vi "Painting_Trajactory_Defalut.vi"(8 "Max-Min Voltage":cluster{"max":dbl, "min":dbl}, 10 "dt":dbl) -> (2 "Waveforms":waveform(dbl)[](graph))   [LabVIEW 2013]
doc: "图片控件可作为用户的绘图界面。本范例主要使用了画笔宽度和样式属性以及子集获取功能。子集获取是指从任意图像中截取一个矩形区域并绘制新图像的功能。"
uses:
  <vilib>/Utility/cursorutil.llb/Set Cursor (Icon Pict).vi
panel:
  in  "清除":bool
  in  "画笔颜色":u32(colorbox)
  in  "停止":bool
  in  "操作":u16(ring)=1 items=["绘制散点", "绘制自由格式线", "绘制直线", "绘制矩形", "选择子集"]
  out "子集":picture
  in  "选择画笔属性":T1={"宽度"=2, "样式"=enum."Solid"}
  out "图片":picture
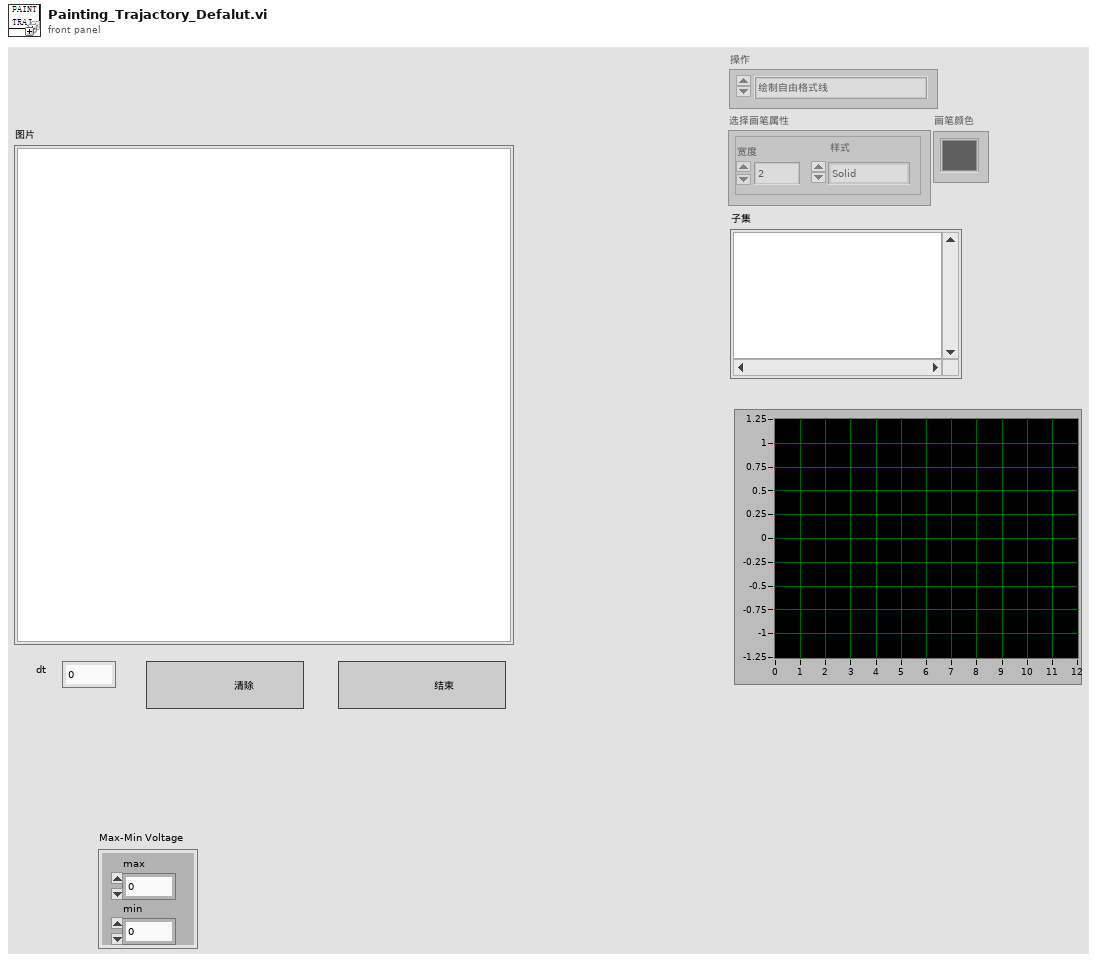
[diagram p1: front panel]
types:
  T1 = cluster{"宽度":u16, "样式":enum32{"Solid", "Dash", "Dot", "DashDot", "DashDotDot"}}
  T2 = enum32{"Solid", "Dash", "Dot", "DashDot", "DashDotDot"}
  T3 = cluster{"Width":u16, "Style":enum32{"Solid", "Dash", "Dot", "DashDot", "DashDotDot"}}
  T4 = enum8{"Enabled", "Disabled", "Disabled and Grayed Out"}
  T5 = typedef "LVMouseTypeDef.ctl" = cluster{"Mouse Position":cluster{"X":i32, "Y":i32}, "Mouse Modifiers":cluster{"Button Down":bool, "Shift Mod":bool, "Menu Mod":bool, "Option Mod":bool}}
  T6 = typedef "imagedata.ctl" = cluster{"image type":i32, "image depth":i32, "image":u8[], "mask":u8[], "colors":u32[], "Rectangle":cluster{"left":i16, "top":i16, "right":i16, "bottom":i16}}
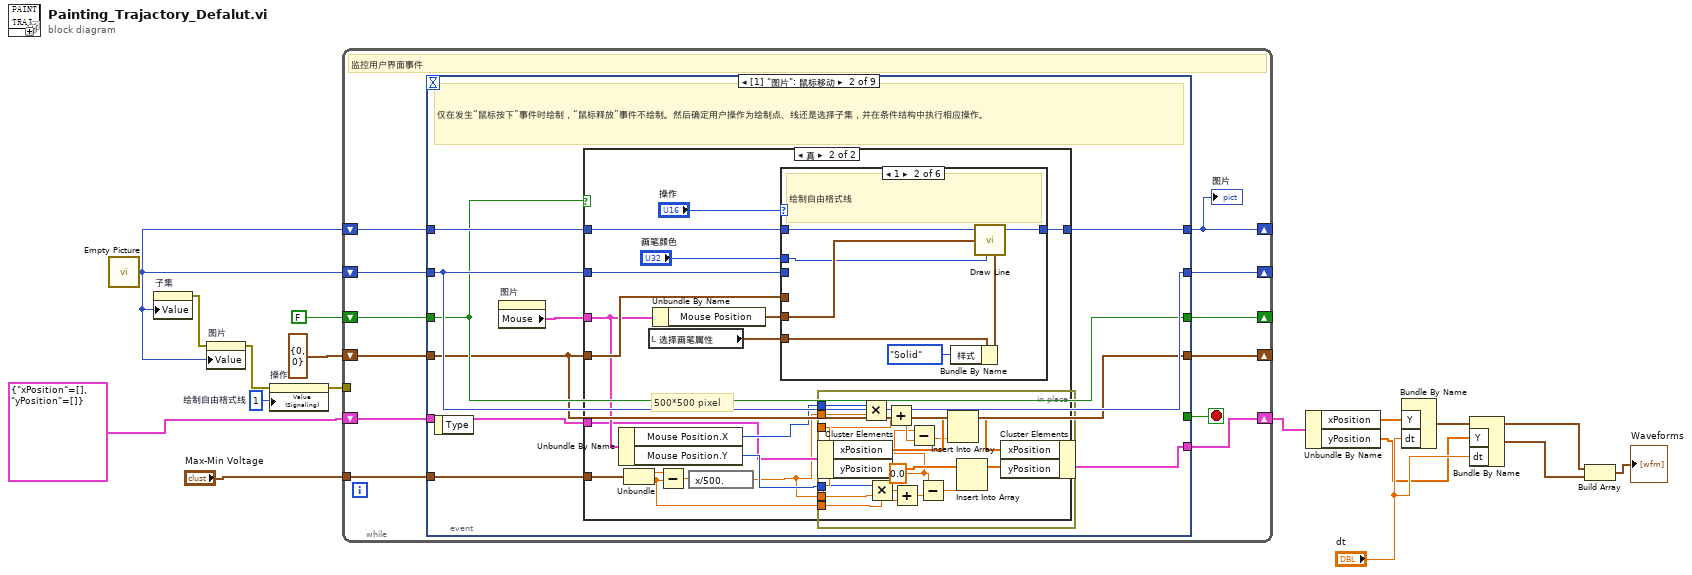
[diagram p0: block diagram]
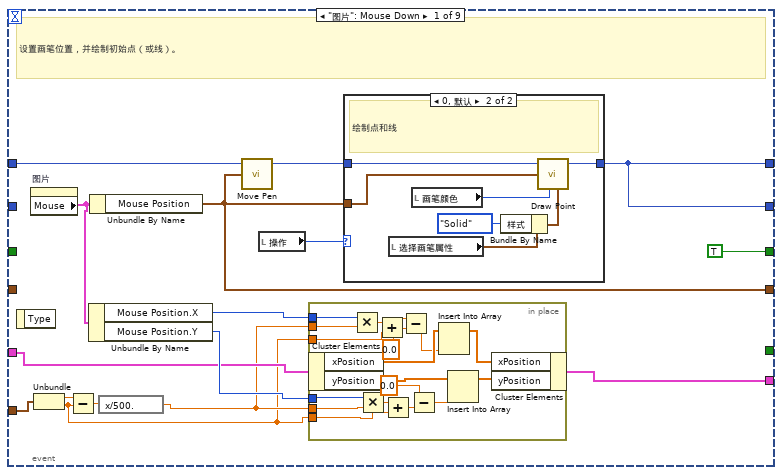
[diagram p2: hidden frame]
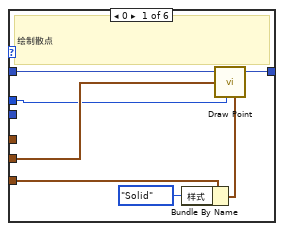
[diagram p5: hidden frame]
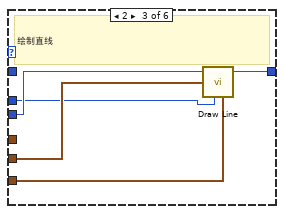
[diagram p6: hidden frame]
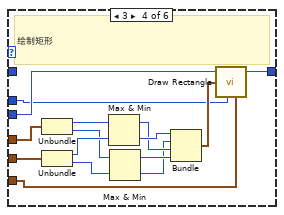
[diagram p7: hidden frame]
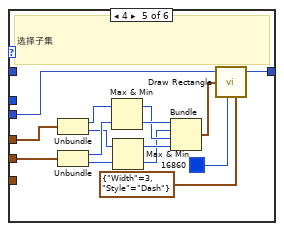
[diagram p8: hidden frame]
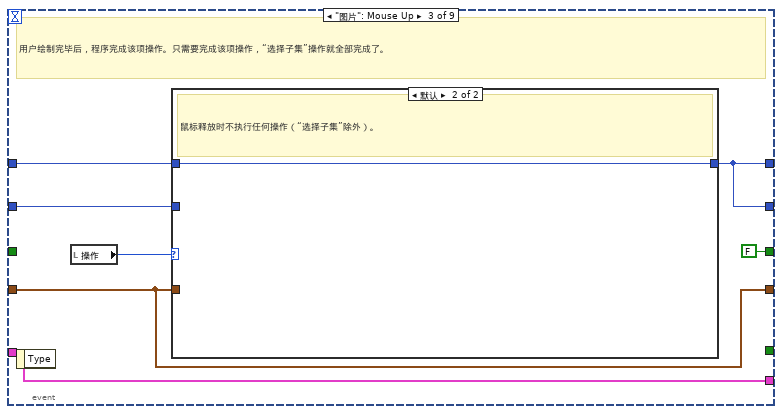
[diagram p10: hidden frame]
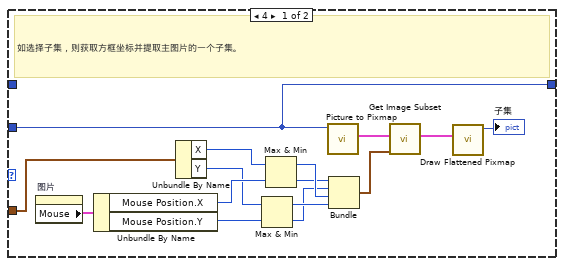
[diagram p11: hidden frame]
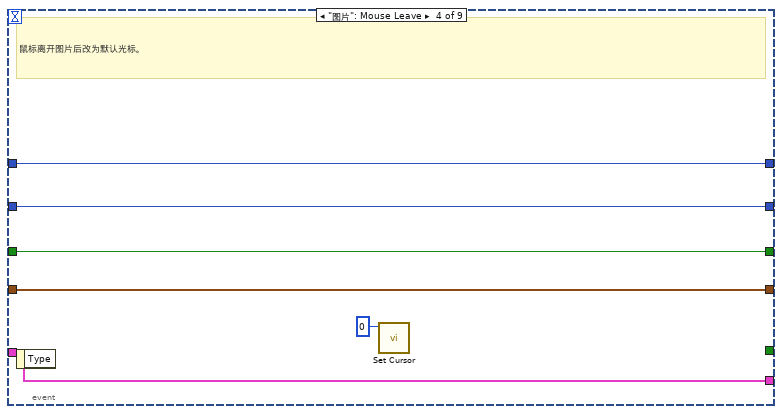
[diagram p12: hidden frame]
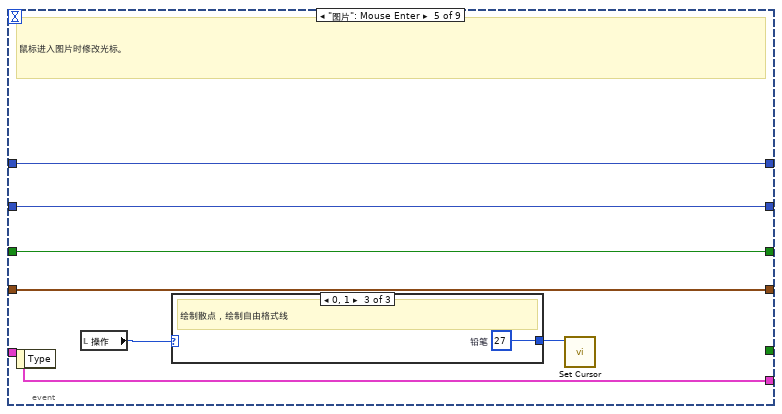
[diagram p13: hidden frame]
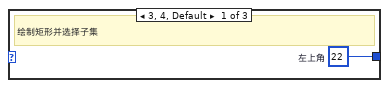
[diagram p14: hidden frame]
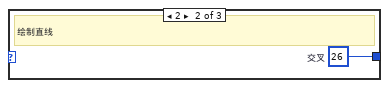
[diagram p15: hidden frame]
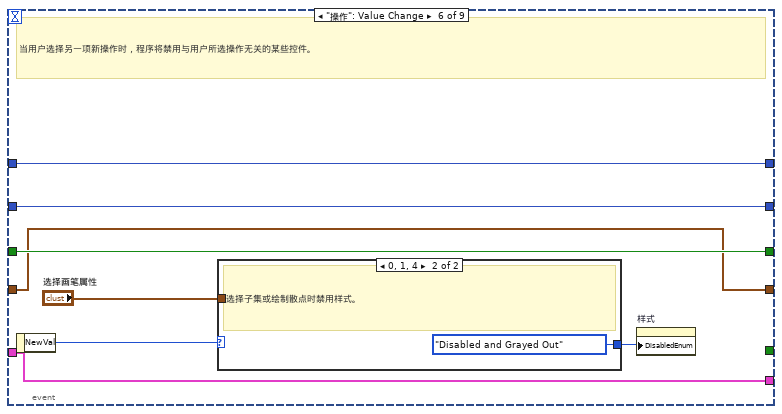
[diagram p16: hidden frame]
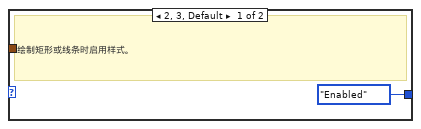
[diagram p17: hidden frame]
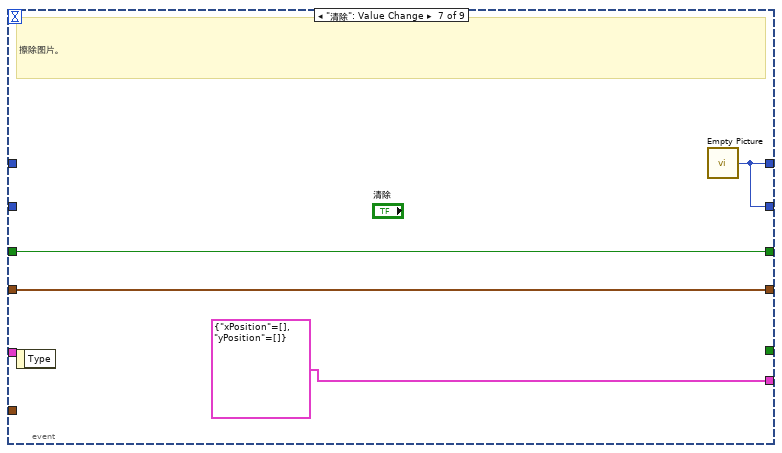
[diagram p18: hidden frame]
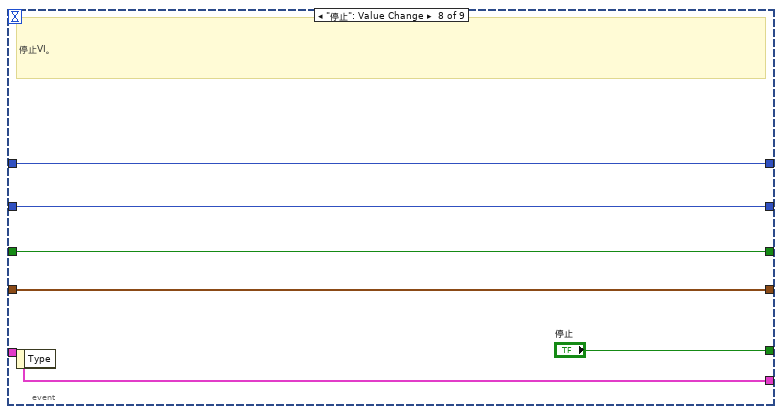
[diagram p19: hidden frame]
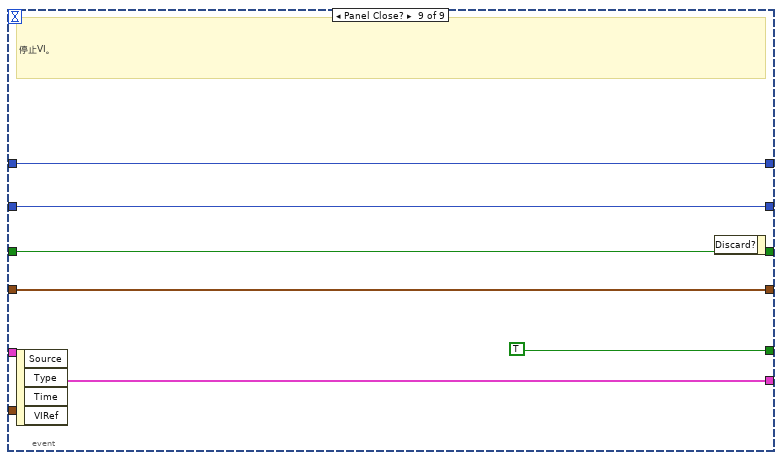
[diagram p20: hidden frame]
diagram:
  w13 = u16 1  # 绘制自由格式线
  n1 = call "Empty Picture"() -> ("empty picture"=w12:picture)
  n2 = property on="子集" class="Pict"("Value"=w12) -> (error out=w14:errorcluster)  [unwired: 2 in, 1 out]
  n3 = property on="图片" class="Pict"(error in=w14, "Value"=w12) -> (error out=w15:errorcluster)  [unwired: 1 in, 1 out]
  n4 = property on="操作" class="Ring (严格)"(error in=w15, "Value (Signaling)"=w13) -> (error out=w16:errorcluster)  [unwired: 1 in, 1 out]
  n5 = while {
    shift-right: [w27] -> _
    shift-left: w12 -> [w26]
    tunnel: w16 -> [_]
    shift-right: [w24] -> _
    shift-left: w12 -> [w25]
    shift-right: [w22] -> _
    shift-left: FALSE -> [w23]
    shift-right: [w20] -> _
    shift-left: cluster{"X":i32, "Y":i32} {"X"=0, "Y"=0} ("Mouse Position") -> [w21]
    shift-right: [w18] -> w6
    shift-left: cluster{"xPosition":dbl[], "yPosition":dbl[]} {"xPosition"=[], "yPosition"=[]} -> [w19]
    tunnel: "Max-Min Voltage" -> [w17]
    stop <- w28 stop-if-true
    # "监控用户界面事件"
    n6 = event shown="[1] \"图片\": 鼠标移动" {
      selector: _ -> [_ _ _ _ _ _ _ _ _]
      dyn-events: _ -> [_ _ _ _ _ _ _ _ _]
      timeout: _ -> [_ _ _ _ _ _ _ _ _]
      tunnel: [_ _ _ _ _ _ _ "停止" TRUE] -> w28
      tunnel: [w42 w78 w170 w194 w201 w212 w219 w224 w231] -> w24
      tunnel: w25 -> [w44 w77 w172 w194 w201 w212 _ w224 w231]
      tunnel: [w42 w76 w170 w195 w202 w211 w219 w223 w230] -> w27
      tunnel: w26 -> [_ w76 w171 w195 w202 w211 _ w223 w230]
      tunnel: w23 -> [_ w75 _ w192 w198 w208 w218 w222 w229]
      tunnel: [TRUE w75 FALSE w192 w198 w208 w218 w222 w229] -> w22
      tunnel: w21 -> [_ w74 w168 w191 w197 w207 w217 w221 w228]
      tunnel: [w39 w74 w168 w191 w197 w207 w217 w221 w228] -> w20
      tunnel: w19 -> [w32 w73 w167 w190 w196 w206 _ w220 w227]
      tunnel: [w29 w72 w167 w190 w196 w206 cluster{"xPosition":i32[], "yPosition":i32[]} {"xPosition"=[], "yPosition"=[]} w220 w227] -> w18
      tunnel: w17 -> [w35 w71 _ _ _ _ _ _ _]
      event "图片": Mouse Down {
        # "设置画笔位置，并绘制初始点（或线）。"
        n7 = event-data() -> ()  [unwired: 1 in, 1 out]
        n8 = property on="图片" class="Pict"() -> ("Mouse"=w38:T5)  [unwired: 2 in, 2 out]
        n9 = Unbundle(w35) -> ("max"=w37:dbl, "min"=w30:dbl)
        n10 = Subtract(x=w37, y=w30) -> (x-y=w36:dbl)
        n11 = Unbundle By Name(w38) -> ("Mouse Position.X"=w34:i32, "Mouse Position.Y"=w33:i32)
        n12 = Unbundle By Name(w38) -> ("Mouse Position"=w39:cluster{"X":i32, "Y":i32})
        n13 = expression code="x/500."(w36) -> (w31:dbl)
        n14 = call <vilib>:"Move Pen.vi"("new position"=w39, "picture"=w44) -> ("new picture"=w43:picture)  [unwired: 3 in]
        n15 = local read "操作"() -> (w41:u16)
        n16 = in-place {
          in-place-border: w33 -> [w53]
          in-place-border: w34 -> [w58]
          in-place-border: w31 -> [w57]
          in-place-border: w30 -> [w51]
          in-place-border: w30 -> [w55]
          in-place-border: w31 -> [w52]
          n17 = in-place-cluster #1(w32) -> ("xPosition"=w62:dbl[], "yPosition"=w60:dbl[])
          n18 = Multiply(x=w58, y=w57) -> (x*y=w56:dbl)
          n19 = Multiply(x=w53, y=w52) -> (x*y=w54:dbl)
          n20 = Add(x=w56, y=w55) -> (x+y=w46:dbl)
          n21 = Add(x=w54, y=w51) -> (x+y=w50:dbl)
          n22 = Subtract(x=0.0, y=w46) -> (x-y=w47:dbl)
          n23 = Subtract(x=0.0, y=w50) -> (x-y=w48:dbl)
          n24 = Insert Into Array(array=w62, new element=w47) -> (w61:dbl[])  [unwired: 1 in]
          n25 = Insert Into Array(array=w60, new element=w48) -> (w59:dbl[])  [unwired: 1 in]
          n26 = in-place-cluster #1("xPosition"=w61, "yPosition"=w59) -> (w29:cluster{"xPosition":dbl[], "yPosition":dbl[]})
        }
        n27 = case shown="0, 默认" w41 {
          tunnel: w43 -> [w63 w70]
          tunnel: [w63 w69] -> w42
          tunnel: w39 -> [_ w68]
          frame 3, 4 {
            # "绘制矩形"
          }
          frame 0, Default {
            # "绘制点和线"
            n28 = local read "选择画笔属性"() -> (w65:T1)
            n29 = local read "画笔颜色"() -> (w67:u32)
            n30 = Bundle By Name(cluster=w65, "样式"=T2."Solid" ("Style")) -> (w64:T1)
            n31 = call <vilib>:"Draw Point.vi"("picture"=w70, "point(x,y)"=w68, "color(black)"=w67, "pen"=w64) -> ("new picture"=w69:picture)  [unwired: 5 in]
          }
        }
      }
      event "图片": Mouse Move {
        # "仅在发生“鼠标按下”事件时绘制，“鼠标释放”事件不绘制。然后确定用户操作为绘制点、线还是选择子集，并在条件结构中执行相应操作。"
        n32 = event-data() -> ()  [unwired: 1 in, 1 out]
        n33 = property on="图片" class="Pict"() -> ("Mouse"=w79:T5)  [unwired: 2 in, 2 out]
        n34 = case shown="真" w75 {
          tunnel: w77 -> [w81 w98]
          tunnel: w79 -> [_ w91]
          tunnel: [w81 w96] -> w78
          tunnel: w76 -> [_ w95]
          tunnel: w74 -> [_ w94]
          tunnel: w73 -> [w80 w88]
          tunnel: [w80 w87] -> w72
          tunnel: w71 -> [_ w86]
          frame False {
          }
          frame True {
            # "500*500 pixel"
            n35 = Unbundle By Name(w91) -> ("Mouse Position.X"=w90:i32, "Mouse Position.Y"=w89:i32)
            n36 = Unbundle(w86) -> ("max"=w85:dbl, "min"=w83:dbl)
            n37 = local read "选择画笔属性"() -> (w93:T1)
            n38 = Unbundle By Name(w91) -> ("Mouse Position"=w97:cluster{"X":i32, "Y":i32})
            n39 = Subtract(x=w85, y=w83) -> (x-y=w84:dbl)
            n40 = expression code="x/500."(w84) -> (w82:dbl)
            n41 = case shown="1" "操作" {
              tunnel: w98 -> [w121 w128 _ _ _ w166]
              tunnel: w94 -> [_ _ _ w149 w164 _]
              tunnel: w97 -> [w122 w129 w134 w150 w165 _]
              tunnel: [w123 w130 w135 w147 w162 w166] -> w96
              tunnel: w95 -> [_ _ w133 w139 w161 _]
              tunnel: w93 -> [w118 w125 w132 w138 _ _]
              tunnel: "画笔颜色" -> [w117 w124 w131 w137 _ _]
              frame 0 {
                # "绘制散点"
                n42 = Bundle By Name(cluster=w118, "样式"=T2."Solid" ("Style")) -> (w120:T1)
                n43 = call <vilib>:"Draw Point.vi"("picture"=w121, "point(x,y)"=w122, "color(black)"=w117, "pen"=w120) -> ("new picture"=w123:picture)  [unwired: 5 in]
              }
              frame 1 {
                # "绘制自由格式线"
                n44 = Bundle By Name(cluster=w125, "样式"=T2."Solid" ("Style")) -> (w126:T1)
                n45 = call <vilib>:"Draw Line.vi"("picture"=w128, "end point"=w129, "color(black)"=w124, "pen"=w126) -> ("new picture"=w130:picture)  [unwired: 5 in]
              }
              frame 2 {
                # "绘制直线"
                n46 = call <vilib>:"Draw Line.vi"("picture"=w133, "end point"=w134, "color(black)"=w131, "pen"=w132) -> ("new picture"=w135:picture)  [unwired: 5 in]
              }
              frame 3 {
                # "绘制矩形"
                n47 = Unbundle(w149) -> ("X"=w146:i32, "Y"=w136:i32)
                n48 = Unbundle(w150) -> ("X"=w145:i32, "Y"=w142:i32)
                n49 = Max & Min(x=w146, y=w145) -> (max(x,y)=w143:i32, min(x,y)=w144:i32)
                n50 = Max & Min(x=w136, y=w142) -> (max(x,y)=w141:i32, min(x,y)=w140:i32)
                n51 = Bundle(w144, w140, w143, w141) -> (w148:cluster{i32, i32, i32, i32})  [unwired: 1 in]
                n52 = call <vilib>:"Draw Rectangle.vi"("picture"=w139, "rect"=w148, "color(black)"=w137, "pen"=w138) -> ("new picture"=w147:picture)  [unwired: 5 in]
              }
              frame 4 {
                # "选择子集"
                n53 = Unbundle(w164) -> ("X"=w160:i32, "Y"=w156:i32)
                n54 = Unbundle(w165) -> ("X"=w159:i32, "Y"=w155:i32)
                n55 = Max & Min(x=w160, y=w159) -> (max(x,y)=w157:i32, min(x,y)=w158:i32)
                n56 = Max & Min(x=w156, y=w155) -> (max(x,y)=w154:i32, min(x,y)=w153:i32)
                n57 = Bundle(w158, w153, w157, w154) -> (w163:cluster{i32, i32, i32, i32})  [unwired: 1 in]
                n58 = call <vilib>:"Draw Rectangle.vi"("picture"=w161, "rect"=w163, "color(black)"=u32 16860, "pen"=T3 {"Width"=3, "Style"=enum."Dash"} ("Select Pen Attributes")) -> ("new picture"=w162:picture)  [unwired: 5 in]
              }
              frame Default {
                # "操作未定义－不执行任何操作。"
              }
            }
            n59 = in-place {
              in-place-border: w89 -> [w107]
              in-place-border: w90 -> [w112]
              in-place-border: w82 -> [w111]
              in-place-border: w83 -> [w105]
              in-place-border: w83 -> [w109]
              in-place-border: w82 -> [w106]
              w100 = 0.0 ("x")
              n60 = in-place-cluster #2(w88) -> ("xPosition"=w116:dbl[], "yPosition"=w114:dbl[])
              n61 = Multiply(x=w112, y=w111) -> (x*y=w110:dbl)
              n62 = Multiply(x=w107, y=w106) -> (x*y=w108:dbl)
              n63 = Add(x=w110, y=w109) -> (x+y=w102:dbl)
              n64 = Add(x=w108, y=w105) -> (x+y=w104:dbl)
              n65 = Subtract(x=w100, y=w102) -> (x-y=w101:dbl)
              n66 = Subtract(x=w100, y=w104) -> (x-y=w103:dbl)
              n67 = Insert Into Array(array=w116, new element=w101) -> (w115:dbl[])  [unwired: 1 in]
              n68 = Insert Into Array(array=w114, new element=w103) -> (w113:dbl[])  [unwired: 1 in]
              n69 = in-place-cluster #2("xPosition"=w115, "yPosition"=w113) -> (w87:cluster{"xPosition":dbl[], "yPosition":dbl[]})
            }
          }
        }
      }
      event "图片": Mouse Up {
        # "用户绘制完毕后，程序完成该项操作。只需要完成该项操作，“选择子集”操作就全部完成了。"
        n70 = event-data() -> ()  [unwired: 1 in, 1 out]
        n71 = local read "操作"() -> (w173:u16)
        n72 = case shown="默认" w173 {
          tunnel: w172 -> [_ w189]
          tunnel: [w183 w189] -> w170
          tunnel: w171 -> [w183 _]
          tunnel: w168 -> [w174 _]
          frame 4 {
            # "如选择子集，则获取方框坐标并提取主图片的一个子集。"
            n73 = property on="图片" class="Pict"() -> ("Mouse"=w187:T5)  [unwired: 2 in, 2 out]
            n74 = Unbundle By Name(w187) -> ("Mouse Position.X"=w177:i32, "Mouse Position.Y"=w175:i32)
            n75 = Unbundle By Name(w174) -> ("X"=w178:i32, "Y"=w176:i32)
            n76 = Max & Min(x=w176, y=w175) -> (max(x,y)=w180:i32, min(x,y)=w179:i32)
            n77 = Max & Min(x=w178, y=w177) -> (max(x,y)=w182:i32, min(x,y)=w181:i32)
            n78 = call <vilib>:"Picture to Pixmap.vi"("picture"=w183) -> ("image data"=w188:T6)  [unwired: 9 in, 1 out]
            n79 = Bundle(w181, w179, w182, w180) -> (w186:cluster{i32, i32, i32, i32})  [unwired: 1 in]
            n80 = call <vilib>:"Get Image Subset.vi"("subset rect"=w186, "image data"=w188) -> ("image subset"=w185:T6)  [unwired: 4 in, 1 out]
            n81 = call <vilib>:"Draw Flattened Pixmap.vi"("image data"=w185) -> ("new picture"=→"子集":picture)  [unwired: 8 in]
          }
          frame Default {
            # "鼠标释放时不执行任何操作（“选择子集”除外）。"
          }
        }
      }
      event "图片": Mouse Leave {
        # "鼠标离开图片后改为默认光标。"
        n82 = event-data() -> ()  [unwired: 1 in, 1 out]
        n83 = call-poly <vilib>:"Set Cursor.vi"("icon"=u16 0) -> ()  [unwired: 9 in, 2 out]
      }
      event "图片": Mouse Enter {
        # "鼠标进入图片时修改光标。"
        n84 = event-data() -> ()  [unwired: 1 in, 1 out]
        n85 = local read "操作"() -> (w199:u16)
        n86 = case shown="0, 1" w199 {
          tunnel: [w203 w204 w205] -> w200
          frame 3, 4, Default {
            w203 = u16 22  # 左上角
            # "绘制矩形并选择子集"
          }
          frame 2 {
            w204 = u16 26  # 交叉
            # "绘制直线"
          }
          frame 0, 1 {
            w205 = u16 27  # 铅笔
            # "绘制散点，绘制自由格式线"
          }
        }
        n87 = call-poly <vilib>:"Set Cursor.vi"("icon"=w200) -> ()  [unwired: 9 in, 2 out]
      }
      event "操作": Value Change {
        # "当用户选择另一项新操作时，程序将禁用与用户所选操作无关的某些控件。"
        n88 = event-data() -> ("NewVal"=w213:u16)  [unwired: 1 in]
        n89 = case shown="0, 1, 4" w213 {
          tunnel: "选择画笔属性" -> [_ _]
          tunnel: [T4."Enabled" ("Disabled") T4."Disabled and Grayed Out" ("Disabled")] -> w209
          frame 2, 3, Default {
            # "绘制矩形或线条时启用样式。"
          }
          frame 0, 1, 4 {
            # "选择子集或绘制散点时禁用样式。"
          }
        }
        n90 = property on="样式" class="Enum (严格)"("DisabledEnum"=w209) -> ()  [unwired: 2 in, 2 out]
      }
      event "清除": Value Change {
        # "擦除图片。"
        n91 = event-data() -> ()  [unwired: 1 in, 1 out]
        n92 = call "Empty Picture"() -> ("empty picture"=w219:picture)
      }
      event "停止": Value Change {
        # "停止VI。"
        n93 = event-data() -> ()  [unwired: 1 in, 1 out]
      }
      event Panel Close? {
        # "停止VI。"
        n94 = event-data() -> ()  [unwired: 1 in, 4 out]
        n95 = event-data() -> ()  [unwired: 2 in, 1 out]
      }
    }
    "图片" <- w24
  }
  n96 = Unbundle By Name(w6) -> ("xPosition"=w8:dbl[], "yPosition"=w1:dbl[])
  n97 = Bundle By Name("Y"=w8, "dt"="dt") -> (w4:waveform(dbl))  [unwired: 1 in]
  n98 = Bundle By Name("Y"=w1, "dt"="dt") -> (w3:waveform(dbl))  [unwired: 1 in]
  n99 = Build Array(w4, w3) -> (→"Waveforms":waveform(dbl)[])
